vi "DEMO.vi"() -> ()   [LabVIEW 2024, in "GRBL 1.1.lvlib"]
doc: "This vi is to help in the implementation of the first project using this tool."
uses:
  GRBL 1.1.lvlib
  Status.ctl
panel:
  out "Numeric":i32
  in  "Z position to go":i32[](array[numeric])=[-10, -20, -5]
  in  "Y position to go":i32[](array[numeric])=[-10, -20, -5]
  in  "X position to go":i32[](array[numeric])=[-10, -20, -5]
  out "Status":T1=enum."Alarm"
  in  "Z-Axis configuration":T2={"Travel resolution\t(step/mm)"=160.0, "Maximum rate\t(mm/min)"=5000, "Acceleration\t(mm/sec^2)"=1000, "Maximum travel\t(mm)"=200}
  in  "Y-Axis configuration":T2={"Travel resolution\t(step/mm)"=160.0, "Maximum rate\t(mm/min)"=5000, "Acceleration\t(mm/sec^2)"=1000, "Maximum travel\t(mm)"=400}
  in  "X-Axis configuration":T2={"Travel resolution\t(step/mm)"=160.0, "Maximum rate\t(mm/min)"=5000, "Acceleration\t(mm/sec^2)"=1000, "Maximum travel\t(mm)"=250}
  out "Version information":string="[VER:1.1f.20170324:]\r\n[OPT:VM,15,128]\r\nok\r\nok\r\n"
  out "Config":string="$0=10\r\n$1=255\r\n$2=0\r\n$3=0\r\n$4=0\r\n$5=1\r\n$6=0\r\n$10=1\r\n$11=0.010\r\n$12=1000.000\r\n$13=0\r\n$20=1\r\n$21=0\r\n$22=1\r\n$23=0\r\n$24=5.000\r\n$25=3000.000\r\n$26=25\r\n$27=2.000\r\n$30=12000\r\n$31=4000\r\n$32=0\r\n$100=13.333\r\n$101=13.333\r\n$102=98.000\r\n$110=50000.000\r\n$111=50000.000\r\n$112=1800.000\r\n$120=250.000\r\n$121=250.000\r\n$122=50.000\r\n$130=267.000\r\n$131=472.000\r\n$132=68.000\r\nok\r\nok\r\n"
  out "error out":errorcluster
  in  "VISA resource name":refnum<visa-resource-name>="COM3"
  # "Set those values in negative from zero"
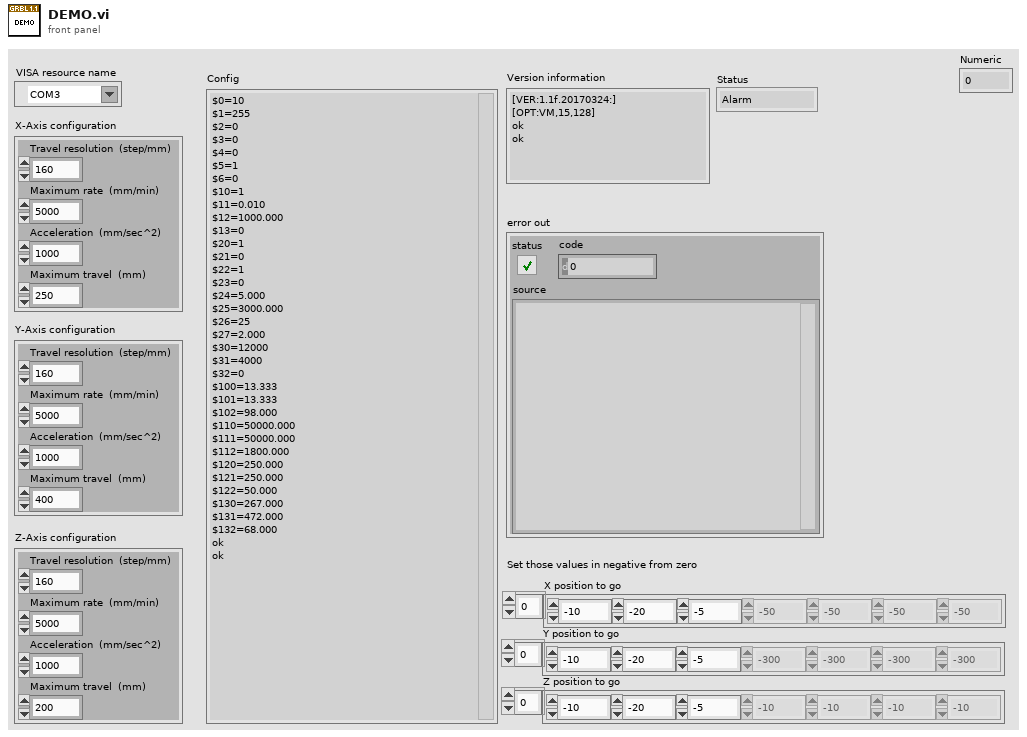
[diagram p1: front panel]
types:
  T1 = typedef "GRBL 1.1.lvlib/Status.ctl" = enum16{"", "Alarm", "Idle", "Run", "Home"}
  T2 = cluster{"Travel resolution\t(step/mm)":sgl, "Maximum rate\t(mm/min)":u32, "Acceleration\t(mm/sec^2)":u32, "Maximum travel\t(mm)":u32}
  T3 = cluster{"Invert enable pin":bool, "Invert limit pin":bool, "Invert probe pin":bool}
  T4 = cluster{"Reverse X":bool, "Reverse Y":bool, "Reverse Z":bool}
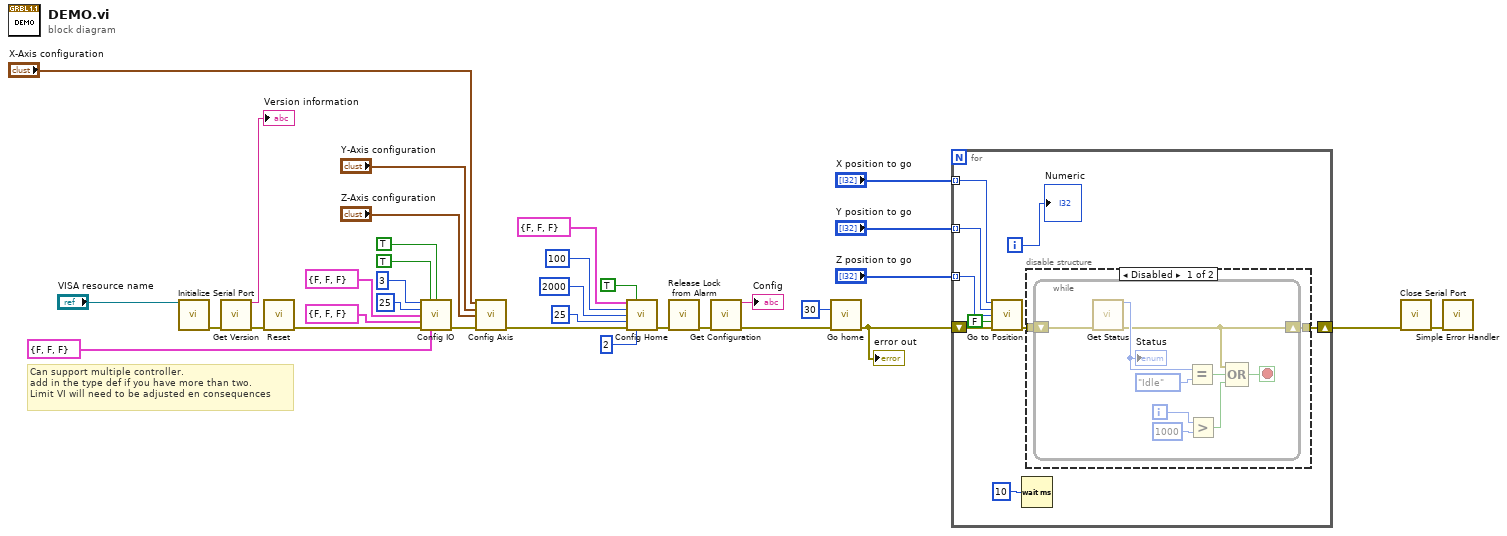
[diagram p0: block diagram]
diagram:
  # "Can support multiple controller.\nadd in the type def if you have more than two.\nLimit VI will need to be adjusted en consequences"
  n1 = call "Initialize Serial Port.vi"("VISA resource name"="VISA resource name") -> ("error out"=w12:errorcluster)  [unwired: 14 in]
  n2 = call "Get Version.vi"("error in (no error)"=w12) -> ("Version information"=→"Version information":string, "error out"=w7:errorcluster)  [unwired: 12 in, 1 out]
  n3 = call "Reset.vi"("error in (no error)"=w7) -> ("error out"=w4:errorcluster)  [unwired: 14 in]
  n4 = call "Config IO.vi"("Pulse time us"=u32 3, "Soft limit enable"=TRUE, "Hard limit enable"=TRUE, "Step idle delay ms (255 keep)"=u8 25, "Step pulse invert"=T4 {"Reverse X"=FALSE, "Reverse Y"=FALSE, "Reverse Z"=FALSE}, "Axis direction"=T4 {"Reverse X"=FALSE, "Reverse Y"=FALSE, "Reverse Z"=FALSE}, "error in (no error)"=w4, "Pins direction"=T3 {"Invert enable pin"=FALSE, "Invert limit pin"=FALSE, "Invert probe pin"=FALSE}) -> ("error out"=w17:errorcluster)  [unwired: 7 in]
  n5 = call "Config Axis.vi"("X-Axis configuration"="X-Axis configuration", "Y-Axis configuration"="Y-Axis configuration", "Z-Axis configuration"="Z-Axis configuration", "error in (no error)"=w17) -> ("error out"=w18:errorcluster)  [unwired: 11 in]
  n6 = call "Config Home.vi"("Homing direction invert"=T4 {"Reverse X"=FALSE, "Reverse Y"=FALSE, "Reverse Z"=FALSE}, "Homing cycle enable"=TRUE, "Homing locate feed rate\tmm/min"=u32 100 ("Homing locate feed rate\tmm/min"), "Homing search seek rate\tmm/min"=u32 2000 ("Homing search seek rate\tmm/min"), "Homing switch debounce delay\tms"=u32 25 ("Homing switch debounce delay\tms"), "error in (no error)"=w18, "Homing switch pull-off distance\tmm"=u32 2 ("Homing switch pull-off distance\tmm")) -> ("error out"=w25:errorcluster)  [unwired: 8 in]
  n7 = call "Release Lock from Alarm.vi"("error in (no error)"=w25) -> ("error out"=w26:errorcluster)  [unwired: 14 in]
  n8 = call "Get Configuration.vi"("error in (no error)"=w26) -> ("Config"=→"Config":string, "error out"=w5:errorcluster)  [unwired: 13 in]
  n9 = call "Go home.vi"("Maximum wait time (45sec)"=30, "error in (no error)"=w5) -> ("error out"=w3:errorcluster)  [unwired: 13 in]
  "error out" <- w3
  n10 = for {
    shift-right: [w43] -> w13
    shift-left: w3 -> [w42]
    tunnel: "X position to go" -> [w41] mode=indexing
    tunnel: "Y position to go" -> [w40] mode=indexing
    tunnel: "Z position to go" -> [w39] mode=indexing
    i -> [w36]
    n11 = call "Go to Position.vi"("X (mm)"=w41, "Y (mm)"=w40, "Z (mm)"=w39, "Wait for finish? (T)"=FALSE, "error in (no error)"=w42) -> ("error out"=w38:errorcluster)  [unwired: 10 in]
    n12 = Wait (ms)(milliseconds to wait=u32 10) -> ()  [unwired: 1 out]
    n13 = disable-structure shown="Disabled" {
      disable-tunnel: [w45 w55] -> w43
      disable-tunnel: w38 -> [w44 w55]
      frame Disabled {
        n14 = while {
          shift-right: [w51] -> w45
          shift-left: w44 -> [w54]
          i -> [w49]
          stop <- w46 stop-if-true
          n15 = call "Get Status.vi"("error in (no error)"=w54) -> ("Status"=w53:T1, "error out"=w51:errorcluster)  [unwired: 10 in, 3 out]
          "Status" <- w53
          n16 = Equal?(x=w53, y=Status."Idle") -> (x = y?=w50:bool)
          n17 = Greater?(x=w49, y=1000) -> (0:w47:bool)
          n18 = Compound Arithmetic op=OR(w51, w50, w47) -> (w46:bool)
        }
      }
      frame Enabled {
      }
    }
    "Numeric" <- w36
  }
  n19 = call "Close Serial Port.vi"("error in (no error)"=w13) -> ("error out"=w1:errorcluster)  [unwired: 14 in]
  n20 = call <vilib>:"Simple Error Handler.vi"("error in (no error)"=w1) -> ()  [unwired: 4 in, 5 out]
